vi "SimpleTCPServer.vi"(11 "port":u16=5001) -> (0 "error out":errorcluster)   [LabVIEW 2014]
doc: "This example VI is to be used in conjunction with the SimpleTCPClient.vi example. \nMake sure to run this example VI prior to running the SimpleTCPClient, otherwise an error will be generated. \n\nBoth the SimpleTCPServer.vi and SimpleTCPClient.vi can run deployed on the Raspberry Pi; the SimpleTCPServer.vi can run deployed on the Raspberry Pi and the SimpleTCPClient.vi remotely on a different networked computer or Raspberry Pi; or the SimpleTCPServer.vi can run remoterly on a different networked computer or Raspberry Pi and the SimpleTCPClient.vi deployed in the Raspberry Pi target.\n\nIf both SimpleTCPServer and SimpleTCPClient run deployed at the same Raspberry Pi, the address control value is to be left unchanged of its default 127.0.0.1 value. If the SimpleTCPClient runs on a different computer than the SimpleTCPServer example, enter the IP address of the computer running the SimpleTCPServer example in the SimpleTCPClient address control.\n\nMake sure the value of the port matches with the port value of the SimpleTCPServer vi.\n\nEnter a string message in the data in control and run the SimpleTPClient VI. Note on the running SimpleTCPServer that the remote address indicator will show the IP address of the computer where SimpleTCPClient ran. The data out indicator of SimpleTCPServer will show the same string value entered in the SimpleTCPClient data in control.\n\nTo stop the SimpleTCPServer execution, enter stop in the data in control and run SimpleTCPClient."
panel:
  out "remote port":u16
  out "remote address":string
  out "data out":string
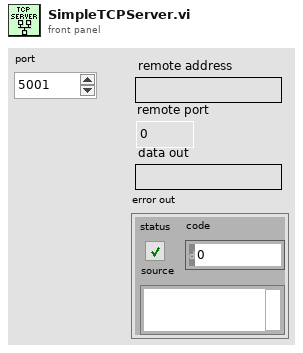
[diagram p1: front panel]
types:
  T1 = enum16{"Standard", "Buffered", "CRLF", "Immediate"}
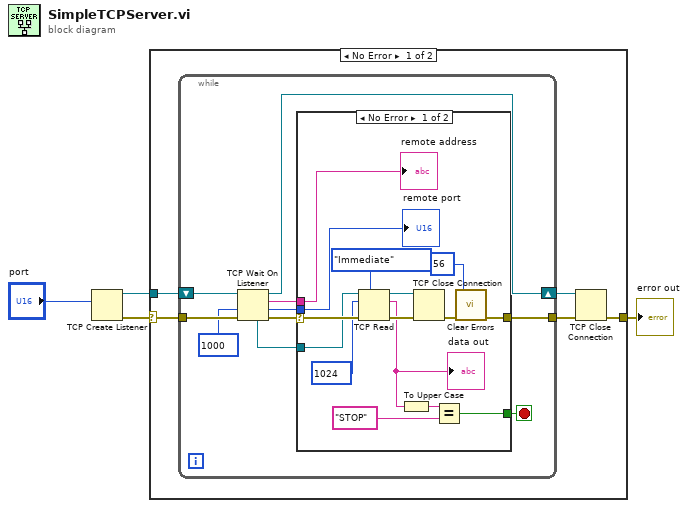
[diagram p0: block diagram]
diagram:
  n1 = TCP Create Listener(10:"port") -> (0:w2:errorcluster, 3:w3:refnum<k5>)  [unwired: 4 in, 1 out]
  n2 = case shown="No Error" w2 {
    selector: w2 -> [w8 w35]
    tunnel: w3 -> [w9 _]
    tunnel: [w5 w35] -> w1
    frame No Error {
      n3 = while {
        shift-right: [w14] -> w6
        shift-left: w9 -> [w19]
        tunnel: w8 -> [w18]
        tunnel: [w11] -> w7
        stop <- w10 stop-if-true
        n4 = TCP Wait On Listener(8:w18, 9:1000 ("timeout ms (wait forever: -1)"), 11:w19) -> (0:w17:errorcluster, 1:w12:u16, 2:w13:string, 3:w14:refnum<k5>, 4:w16:refnum<k5>)  [unwired: 1 in]
        n5 = case shown="No Error" w17 {
          selector: w17 -> [w34 _]
          tunnel: w16 -> [w33 _]
          tunnel: w13 -> [w26 _]
          tunnel: w12 -> [w25 _]
          tunnel: [w21 _] -> w11
          tunnel: [w27 _] -> w10
          frame No Error {
            n6 = TCP Read(connection ID=w33, bytes to read=1024, error in (no error)=w34, 7:T1."Immediate" ("mode (standard)")) -> (connection ID out=w31:refnum<k5>, data out=w30:string, error out=w32:errorcluster)  [unwired: 1 in]
            "data out" <- w30
            n7 = To Upper Case(1:w30) -> (0:w29:string)
            n8 = TCP Close Connection(connection ID=w31, error in (no error)=w32) -> (error out=w22:errorcluster)  [unwired: 1 in, 1 out]
            n9 = Equal?(x=w29, y="STOP") -> (x = y?=w27:bool)
            n10 = call <vilib>:"Clear Errors.vi"("error in (no error)"=w22, "specific error code to clear (0: all)"=56) -> ("error out"=w21:errorcluster)  [unwired: 4 in, 1 out]
            "remote address" <- w26
            "remote port" <- w25
          }
          frame Error {
          }
        }
      }
      n11 = TCP Close Connection(connection ID=w6, error in (no error)=w7) -> (error out=w5:errorcluster)  [unwired: 1 in, 1 out]
    }
    frame Error {
    }
  }
  "error out" <- w1
